vi "Configure Pulse (Transistion).vi"(8 "error in (no error)":errorcluster, 10 "Transition Time (10e-9 s)":dbl=1e-08, 11 "VISA resource name":refnum<visa-resource-name>) -> (0 "error out":errorcluster, 3 "VISA resource name out":refnum<visa-resource-name>)   [LabVIEW 2017, in "Keithley 3390.lvlib"]
doc: "Sets the pulse edge transtion time of the pulse waveform."
uses:
  Keithley 3390.lvlib
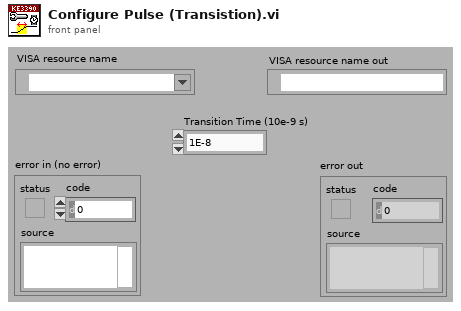
[diagram p1: front panel]
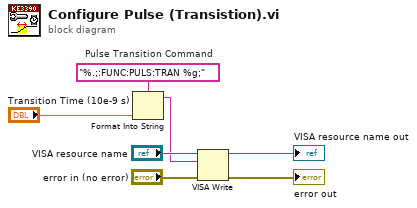
[diagram p0: block diagram]
diagram:
  w5 = "%.;:FUNC:PULS:TRAN %g;"  # Pulse Transition Command
  n1 = Format Into String(format string=w5, "Transition Time (10e-9 s)") -> (resulting string=w3:string)  [unwired: 2 in, 1 out]
  n2 = VISA Write(VISA resource name="VISA resource name", write buffer=w3, error in (no error)="error in (no error)") -> (VISA resource name out=→"VISA resource name out":refnum<visa-resource-name>, error out=→"error out":errorcluster)  [unwired: 1 out]
